vi "Configure Spectrum Emission Mask (Offset Level).vi"(0 "VISA resource name":refnum<visa-resource-name>, 5 "SEM Level Offset":i32[](array[ring]) items=["Off", "On"], 7 "SEM Level":dbl[](array[numeric]) min=-120.0 max=50.0 format="%.2f", 9 "SEM Attenuator Offset":i32[](array[ring]) items=["Off", "On"], 11 "error in (no error)":errorcluster, 12 "SEM Attenuator":i32[](array[numeric]) min=0 max=60) -> (4 "VISA resource name out":refnum<visa-resource-name>, 15 "error out":errorcluster)   [LabVIEW 2020, in "Anritsu Signal Analyzer Series.lvlib"]
doc: "Configures the setup for offset level of SEM measurement settings of the spectrum analyzer."
uses:
  Anritsu Signal Analyzer Series.lvlib
panel:
  # "dBm"
  # "dB"
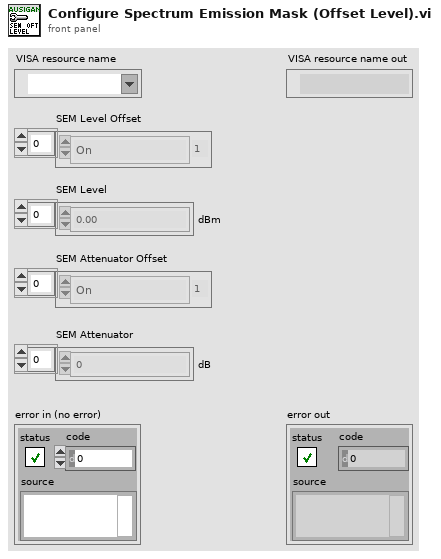
[diagram p1: front panel]
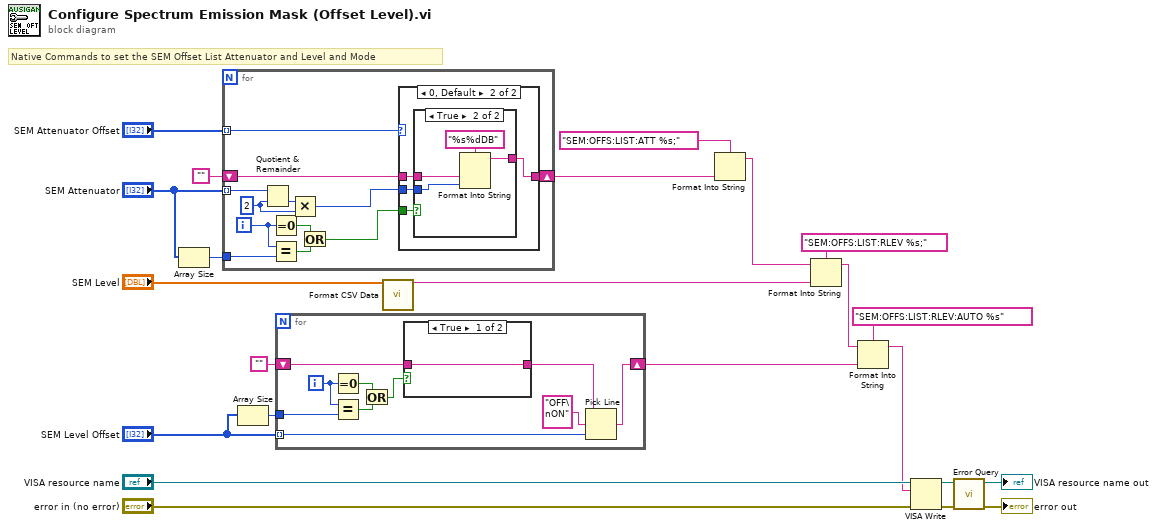
[diagram p0: block diagram]
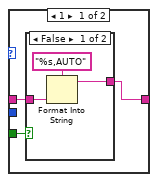
[diagram p2: hidden frame]
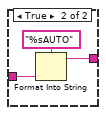
[diagram p3: hidden frame]
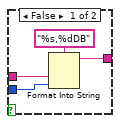
[diagram p4: hidden frame]
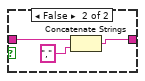
[diagram p5: hidden frame]
diagram:
  # "Native Commands to set the SEM Offset List Attenuator and Level and Mode"
  n1 = Array Size(array="SEM Attenuator") -> (size(s)=w3:i32)
  n2 = for {
    shift-right: [w32] -> w11
    shift-left: "" ("Empty String Constant") -> [w33]
    tunnel: "SEM Attenuator" -> [w31] mode=indexing
    tunnel: w3 -> [w27]
    tunnel: "SEM Attenuator Offset" -> [w25] mode=indexing
    i -> [w28]
    w34 = 2
    n3 = Quotient & Remainder(x=w31, y=w34) -> (floor(x/y)=w35:i32)  [unwired: 1 out]
    n4 = Equal To 0?(x=w28) -> (x = 0?=w29:bool)
    n5 = Equal?(x=w28, y=w27) -> (x = y?=w30:bool)
    n6 = Multiply(x=w35, y=w34) -> (x*y=w24:i32)
    n7 = Or(x=w29, y=w30) -> (x .or. y?=w26:bool)
    n8 = case shown="0, Default" w25 {
      tunnel: w33 -> [w38 w48]
      tunnel: [w37 w47] -> w32
      tunnel: w24 -> [_ w46]
      tunnel: w26 -> [w36 w45]
      frame 1 {
        n9 = case shown="False" w36 {
          tunnel: w38 -> [w40 w42]
          tunnel: [w39 w44] -> w37
          frame False {
            n10 = Format Into String(format string="%s,AUTO" ("Format String"), w40) -> (resulting string=w39:string)  [unwired: 2 in, 1 out]
          }
          frame True {
            n11 = Format Into String(format string="%sAUTO", w42) -> (resulting string=w44:string)  [unwired: 2 in, 1 out]
          }
        }
      }
      frame 0, Default {
        n12 = case shown="True" w45 {
          tunnel: w46 -> [w50 w53]
          tunnel: w48 -> [w51 w54]
          tunnel: [w49 w56] -> w47
          frame False {
            n13 = Format Into String(format string="%s,%dDB" ("Format String"), w51, w50) -> (resulting string=w49:string)  [unwired: 2 in, 1 out]
          }
          frame True {
            n14 = Format Into String(format string="%s%dDB", w54, w53) -> (resulting string=w56:string)  [unwired: 2 in, 1 out]
          }
        }
      }
    }
  }
  n15 = Array Size(array="SEM Level Offset") -> (size(s)=w4:i32)
  n16 = for {
    shift-right: [w58] -> w14
    shift-left: "" ("Empty String Constant") -> [w66]
    tunnel: "SEM Level Offset" -> [w57] mode=indexing
    tunnel: w4 -> [w61]
    i -> [w63]
    n17 = Equal To 0?(x=w63) -> (x = 0?=w64:bool)
    n18 = Equal?(x=w63, y=w61) -> (x = y?=w65:bool)
    n19 = Or(x=w64, y=w65) -> (x .or. y?=w62:bool)
    n20 = case shown="True" w62 {
      tunnel: w66 -> [w67 w70]
      tunnel: [w67 w68] -> w59
      frame True {
      }
      frame False {
        n21 = Concatenate Strings(w70, "," ("string")) -> (w68:string)
      }
    }
    n22 = Pick Line(string ("")=w59, multi-line string="OFF\nON" ("複数行文字列"), line index=w57) -> (output string=w58:string)
  }
  n23 = call "Format CSV Data.vi"("Data_In"="SEM Level") -> ("Data_out"=w8:string)  [unwired: 14 in]
  n24 = Format Into String(format string="SEM:OFFS:LIST:ATT %s;" ("_CommandSet"), w11) -> (resulting string=w7:string)  [unwired: 2 in, 1 out]
  n25 = Format Into String(format string="SEM:OFFS:LIST:RLEV %s;" ("_CommandSet"), initial string=w7, w8) -> (resulting string=w6:string)  [unwired: 1 in, 1 out]
  n26 = Format Into String(format string="SEM:OFFS:LIST:RLEV:AUTO %s" ("_CommandSet"), initial string=w6, w14) -> (resulting string=w5:string)  [unwired: 1 in, 1 out]
  n27 = VISA Write(VISA resource name="VISA resource name", write buffer=w5, error in (no error)="error in (no error)") -> (VISA resource name out=w2:refnum<visa-resource-name>, error out=w1:errorcluster)  [unwired: 1 out]
  n28 = call "Error Query.vi"("error in (no error)"=w1, "VISA resource name"=w2) -> ("error out"=→"error out":errorcluster, "VISA resource name out"=→"VISA resource name out":refnum<visa-resource-name>)  [unwired: 6 in, 2 out]
